vi "Begin.vi"(8 "error in":errorcluster) -> (0 "error out":errorcluster)   [LabVIEW 2019]
doc: "Called before other user functions, this VI is expected to open initial I/O refnums, load in file data, and do all program initialization. Notice that the <B>error out</B> terminal is simply used for data flow. Wiring it to other structures or subVIs ensures that this VI runs first."
uses:
  <vilib>/Rock Robotics/SystemInterfaces/i2clib/i2c_bus.ctl
  <vilib>/Rock Robotics/WPI/DriverStation/WPI_DriverStationRobotMode2.ctl
  <vilib>/Rock Robotics/WPI/Joystick/WPI_JoystickDeviceEnum.ctl
  <vilib>/Rock Robotics/WPI/SafetyOutput/WPI_SafetyOutputConfigMenu.ctl
  <vilib>/Rock Robotics/WPI/ThirdParty/Phoenix-LabVIEW/Motor Controller/Controls/CTRE_Phoenix_MotorControl_ControlMode.ctl
  <vilib>/Rock Robotics/WPI/ThirdParty/Phoenix-LabVIEW/Motor Controller/Controls/CTRE_Phoenix_MotorControl_FeedbackDevice.ctl
  <vilib>/Rock Robotics/WPI/Solenoid/WPI_SolenoidChannel.ctl
  <vilib>/Rock Robotics/WPI/ThirdParty/Phoenix-LabVIEW/Motor Controller/Controls/CTRE_Phoenix_MotorControl_NeutralMode.ctl
  <vilib>/Rock Robotics/WPI/ThirdParty/REV Robotics/SPARK MAX/Typedef/Spark MAX Motor Type.ctl
  <vilib>/Rock Robotics/WPI/ThirdParty/Phoenix-LabVIEW/Motor Controller/Controls/CTRE_Phoenix_MotorControl_FeedbackDevice_TalonFX.ctl
  <vilib>/Rock Robotics/WPI/ThirdParty/Phoenix-LabVIEW/Motor Controller/Controls/CTRE_Phoenix_MotorControl_VelocityMeasurementPeriod.ctl
  <vilib>/Rock Robotics/SystemInterfaces/DIO/FPGA_DIOChannel.ctl
  <vilib>/Rock Robotics/WPI/ThirdParty/REV Robotics/SPARK MAX/Typedef/Spark MAX Control Type.ctl
  Robot Global Data.vi
  <vilib>/Rock Robotics/Network Tables/NT Write String Array.vi
  <vilib>/Rock Robotics/WPI/Solenoid/WPI_SolenoidOpenDouble.vi
  <vilib>/Rock Robotics/WPI/RobotDrive/WPI_RobotDriveOpen4MotorWithExistingMotors.vi
panel:
  in  "Blue Calibration":cluster{"R":dbl, "G":dbl, "B":dbl}={"R"=0.143, "G"=0.427, "B"=0.429}
  in  "Green Calibration":cluster{"R":dbl, "G":dbl, "B":dbl}={"R"=0.197, "G"=0.561, "B"=0.24}
  in  "Red Calibration":cluster{"R":dbl, "G":dbl, "B":dbl}={"R"=0.561, "G"=0.323, "B"=0.114}
  in  "Yellow Calibration":cluster{"R":dbl, "G":dbl, "B":dbl}={"R"=0.361, "G"=0.524, "B"=0.113}
  in  "I2C Bus":T1
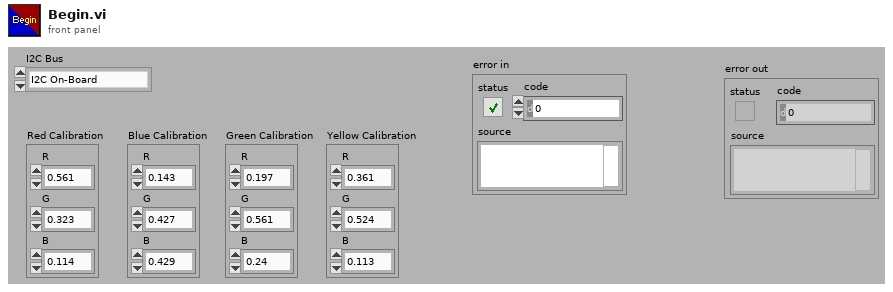
[diagram p1: front panel]
types:
  T1 = typedef "i2c_bus.ctl" = enum16{"I2C On-Board", "I2C MXP", "Invalid"}
  T2 = cluster{"P Gain":dbl, "I Gain":dbl, "D Gain":dbl, "F Gain":dbl, "I Zone":dbl, "Min Output":dbl, "Max Output":dbl}
  T3 = typedef "Spark MAX Motor Type.ctl" = enum16{"Brushed", "Brushless"}
  T4 = typedef "Spark MAX Control Type.ctl" = enum16{"Percent VBus", "Voltage", "Velocity", "Position", "Smart Motion", "Current", "Smart Velocity"}
  T5 = typedef "CTRE_Phoenix_MotorControl_NeutralMode.ctl" = enum8{"EEPROMSetting", "Override to Coast", "Override to Brake"}
  T6 = typedef "WPI_SolenoidChannel.ctl" = enum8{"Solenoid 0", "Solenoid 1", "Solenoid 2", "Solenoid 3", "Solenoid 4", "Solenoid 5", "Solenoid 6", "Solenoid 7", "Invalid"}
  T7 = typedef "FPGA_DIOChannel.ctl" = enum8{"DIO 0", "DIO 1", "DIO 2", "DIO 3", "DIO 4", "DIO 5", "DIO 6", "DIO 7", "DIO 8", "DIO 9", "DIO MXP 0", "DIO MXP 1", "DIO MXP 2", "DIO MXP 3", "DIO MXP 4", "DIO MXP 5", "DIO MXP 6", "DIO MXP 7", "DIO MXP 8", "DIO MXP 9", "DIO MXP 10", "DIO MXP 11", "DIO MXP 12", "DIO MXP 13", "DIO MXP 14", "DIO MXP 15", "SPI Port CS1", "SPI Port CS2", "SPI Port CS3", "SPI Port MISO", "SPI Port MOSI", "Invalid"}
  T8 = typedef "CTRE_Phoenix_MotorControl_VelocityMeasurementPeriod.ctl" = u16
  T9 = typedef "CTRE_Phoenix_MotorControl_FeedbackDevice_TalonFX.ctl" = i8
  T10 = typedef "CTRE_Phoenix_MotorControl_ControlMode.ctl" = u16
  T11 = typedef "CTRE_Phoenix_MotorControl_FeedbackDevice.ctl" = i8
  T12 = typedef "WPI_SafetyOutputConfigMenu.ctl" = enum16{"Enable", "Disable"}
  T13 = typedef "WPI_JoystickDeviceEnum.ctl" = enum16{"USB 0", "USB 1", "USB 2", "USB 3", "USB 4", "USB 5"}
  T14 = typedef "WPI_DriverStationRobotMode2.ctl" = enum16{"Autonomous Disabled", "Autonomous Enabled", "Teleop Disabled", "Teleop Enabled", "Disconnected", "Finish", "Test Disabled", "Test Enabled", "Emergency Stopped"}
  T15 = typedef "Color Sensor V3 DevRef.ctl" = cluster{"I2CDevRef":T16}
  T16 = typedef "WPI_I2CDevRef.ctl" = cluster{"DevStatus":errorcluster, "Device Address":u8, "Handle":i32, "I2C Bus":T1}
  T17 = typedef "WPI_JoystickDevRef.ctl" = cluster{"Device":T13}
  T18 = typedef "WPI_DigitalInputDevRef.ctl" = cluster{"DevStatus":errorcluster, "DIO Channel":T7}
  T19 = typedef "WPI_MotorControlDeviceRef.ctl" = cluster{"DeviceStatus":errorcluster, "Type":T20, "PWM":cluster{"PWM Channel":T21, "DeadBand":T22}, "CAN":cluster{"Device Number":u8, "SetOutput VI Ref":variant, "GetOutput VI Ref":variant, "Enable VI Ref":variant, "Disable VI Ref":variant, "Data":variant}, "Invert":bool, "DIO PWM":cluster{"PWM \"Enable\" Channel":T21, "DIOChannel":T7, "PWM Rate":dbl}}
  T20 = typedef "WPI_MotorControlType.ctl" = enum16{"PWM", "CAN", "DIO PWM"}
  T21 = typedef "FPGA_DIOPWMChannel.ctl" = enum8{"PWM 0", "PWM 1", "PWM 2", "PWM 3", "PWM 4", "PWM 5", "PWM 6", "PWM 7", "PWM 8", "PWM 9", "PWM MXP 0", "PWM MXP 1", "PWM MXP 2", "PWM MXP 3", "PWM MXP 4", "PWM MXP 5", "PWM MXP 6", "PWM MXP 7", "PWM MXP 8", "PWM MXP 9", "Invalid"}
  T22 = typedef "WPI_PWMDeadband.ctl" = cluster{"Name":string, "maxPositivePwm":i32, "minPositivePwm":i32, "centerPwm":i32, "maxNegativePwm":i32, "minNegativePwm":i32, "angularRange":u16}
  T23 = typedef "WPI_SolenoidDevRef.ctl" = cluster{"DevStatus":errorcluster, "Pneumatics Control Module":u8, "Forward Solenoid Channel":T6, "Reverse Solenoid Channel":T6}
  T24 = typedef "WPI_RobotDriveDevRef.ctl" = cluster{"DevStatus":errorcluster, "Motors[]":T19[], "Square Inputs":bool, "Max Output":dbl}
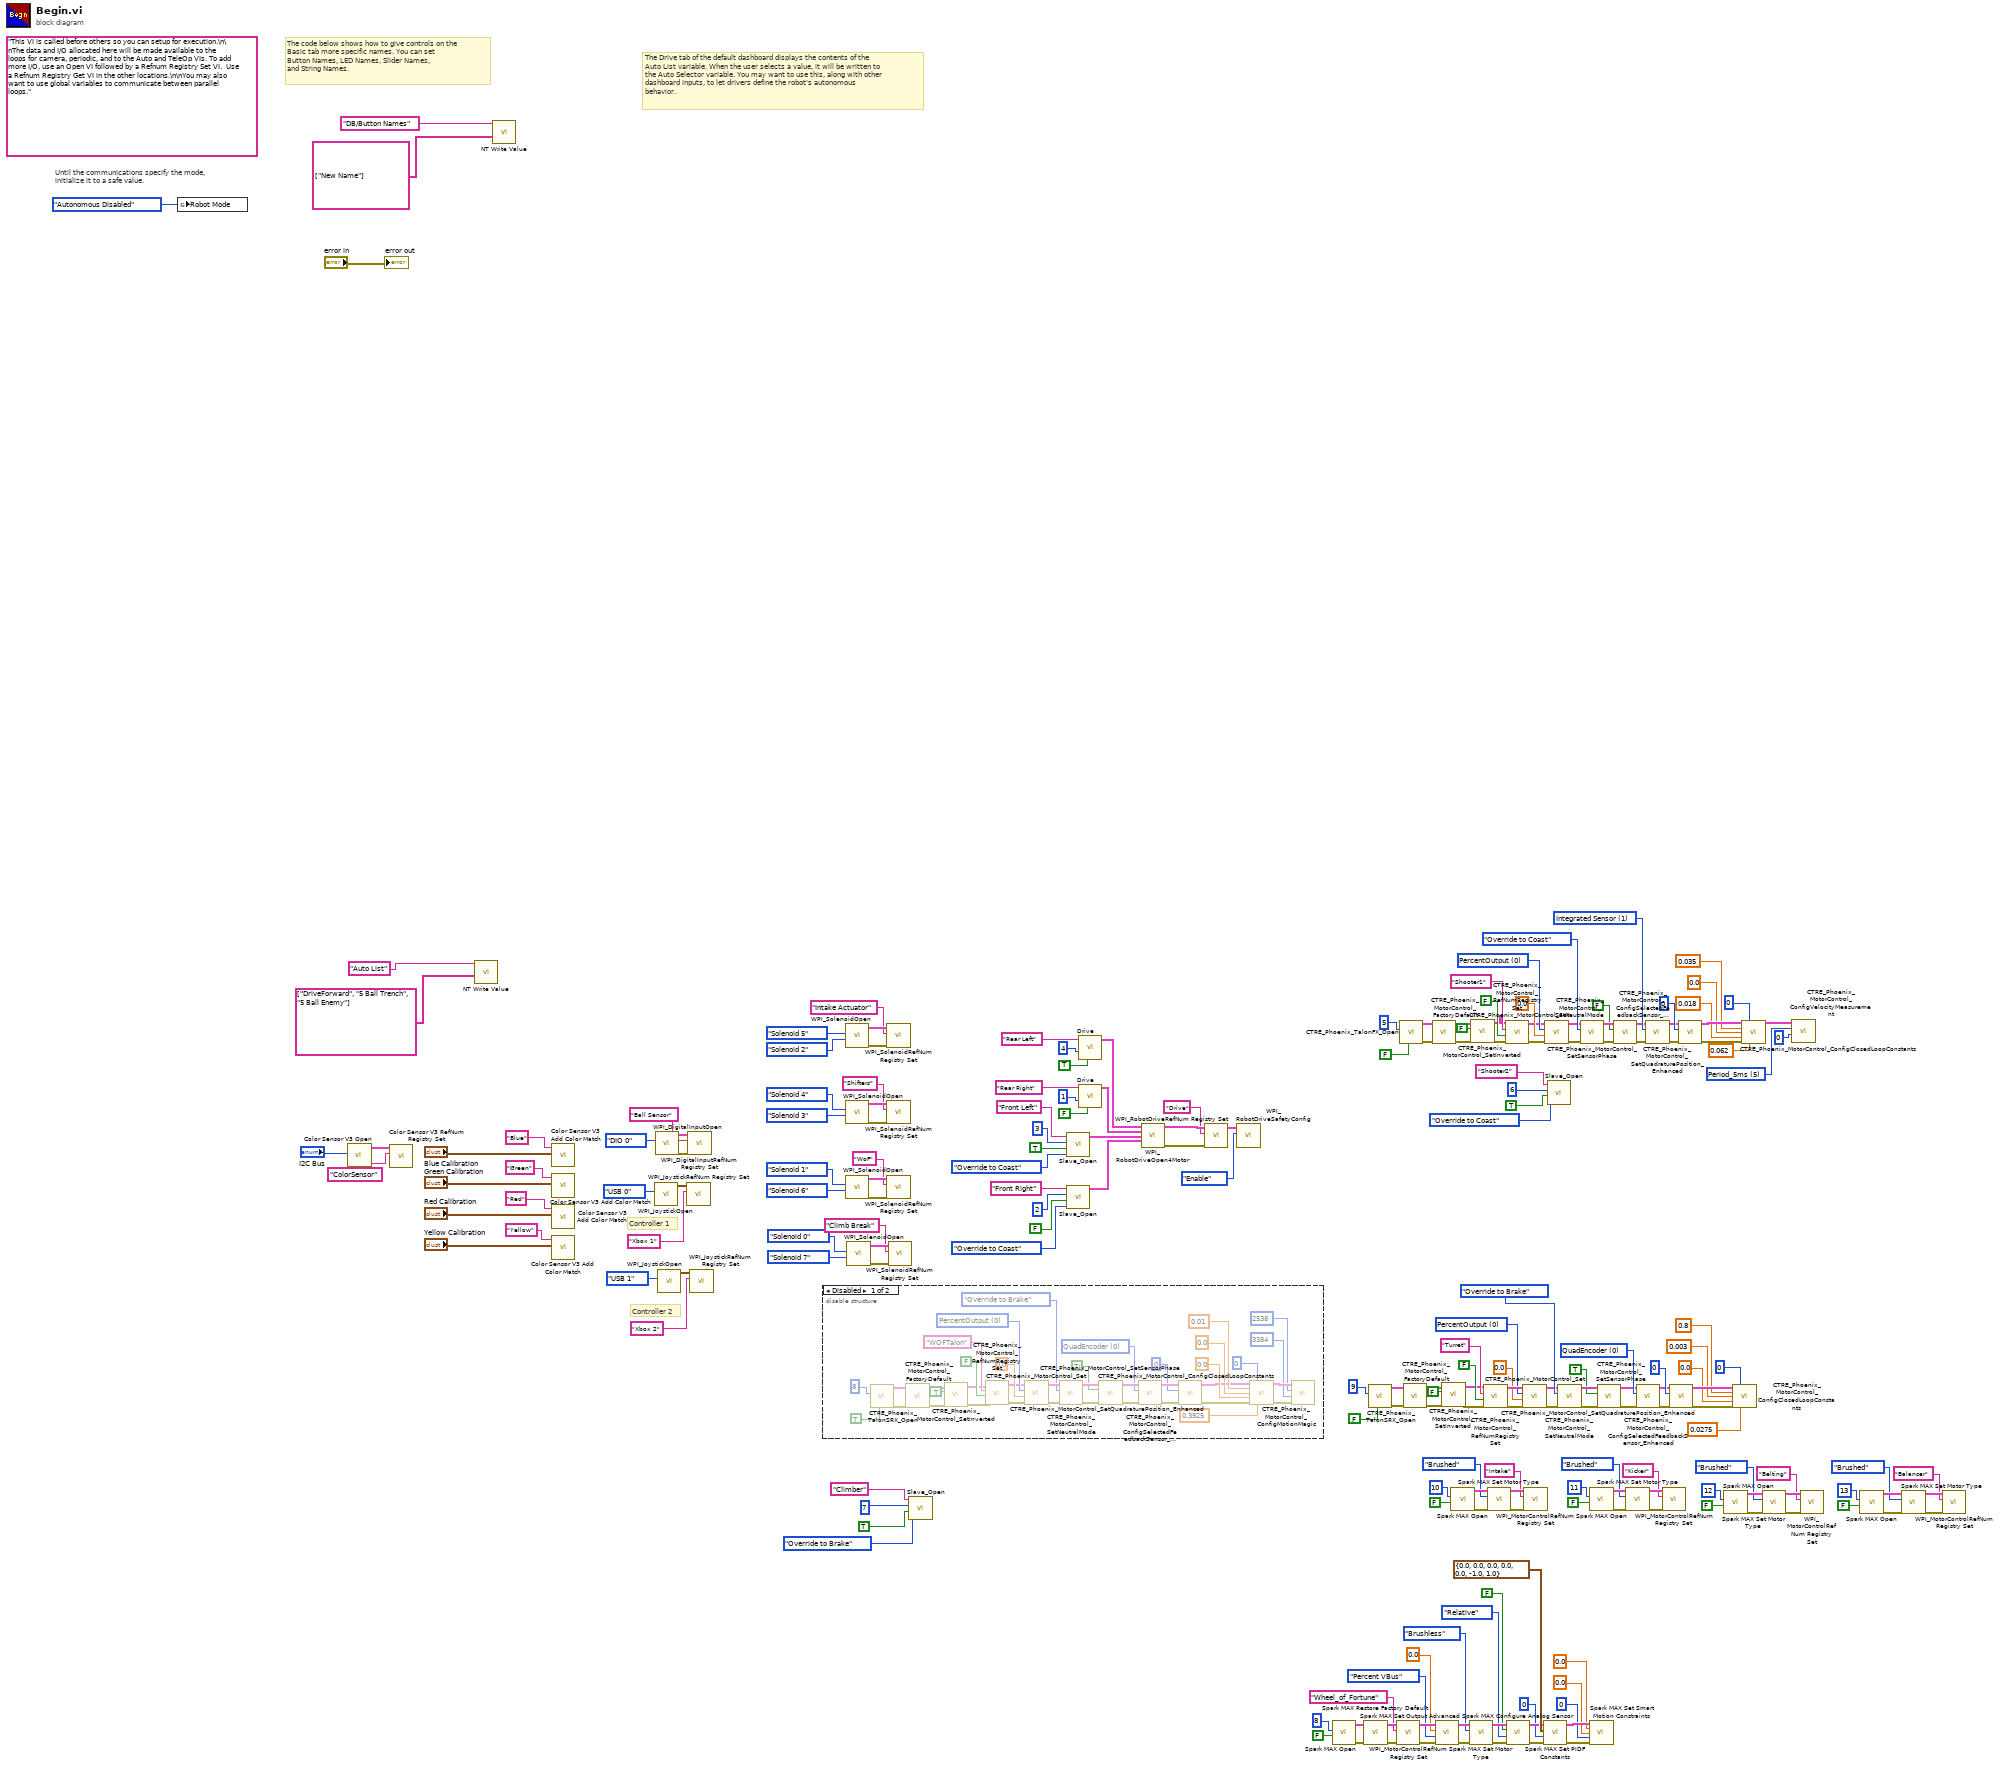
[diagram p0: block diagram]
diagram:
  w123 = T8 5 items=["Period_1ms"=1, "Period_2ms"=2, "Period_5ms"=5, "Period_10ms"=10, "Period_20ms"=20, "Period_25ms"=25, "Period_50ms"=50, "Period_100ms"=100] ("Velocity Measurement Period")
  w113 = T9 1 items=["Integrated Sensor"=1, "Sensor Sum (S0 + S1)"=9, "Sensor Difference (D0 - D1)"=10, "Remote Source 0"=11, "Remote Source 1"=12, "None"=14, "Software Emulated"=15] ("Talon FX Feedback Device")
  w111 = T10 0 items=["PercentOutput"=0, "Position"=1, "Velocity"=2, "Current"=3, "Follower"=5, "MotionProfile"=6, "MotionMagic"=7, "MotionProfileArc"=10, "Disabled"=15] ("Control Mode")
  w166 = T11 0 items=["None"=-1, "QuadEncoder"=0, "Analog"=2, "Tachometer"=4, "Pulse Width Encoded Position"=8, "Sensor Sum (S0 + S1)"=9, "Sensor Difference (D0 - D1)"=10, "Remote Source 0"=11, "Remote Source 1"=12, "Software Emulated"=15] ("Feedback Device")
  w171 = T10 0 items=["PercentOutput"=0, "Position"=1, "Velocity"=2, "Current"=3, "Follower"=5, "MotionProfile"=6, "MotionMagic"=7, "MotionMagicArc"=8, "MotionProfileArc"=10, "Disabled"=15] ("Control Mode")
  (unwired) "This VI is called before others so you can setup for execution.\n\nThe data and I/O allocated here will be made available to the loops for camera, periodic, and to the Auto and TeleOp VIs. To add more I/O, use an Open VI followed by a Refnum Registry Set VI.  Use a Refnum Registry Get VI in the other locations.\n\nYou may also want to use global variables to communicate between parallel loops."
  # "Controller 2"
  # "Controller 1"
  # "The Drive tab of the default dashboard displays the contents of the\nAuto List variable. When the user selects a value, it will be written to\nthe Auto Selector variable. You may want to use this, along with other\ndashboard inputs, to let drivers define the robot's autonomous\nbehavior."
  # "The code below shows how to give controls on the\nBasic tab more specific names. You can set\nButton Names, LED Names, Slider Names,\nand String Names."
  # "Until the communications specify the mode,\ninitialize it to a safe value."
  n1 = global write "Robot Global Data.vi" "Robot Mode"(WPI_DriverStationRobotMode2."Autonomous Disabled" ("Robot Mode")) -> ()
  n2 = call <vilib>:"Color Sensor V3 Open.vi"("I2C Bus"="I2C Bus") -> ("ColorSensorDevRef"=w190:T15)  [unwired: 9 in, 1 out]
  n3 = call <vilib>:"Color Sensor V3 RefNum Registry Set.vi"("refnum name"="ColorSensor", "ColorSensorDevRef"=w190) -> ()  [unwired: 8 in, 2 out]
  n4 = call-poly <vilib>:"NT Write Value.vi"("String Array"=string[] ["DriveForward", "5 Ball Trench", "5 Ball Enemy"], "Name"="Auto List") -> ()  [unwired: 9 in, 1 out]
  n5 = call-poly <vilib>:"NT Write Value.vi"("String Array"=string[] ["New Name"], "Name"="DB/Button Names") -> ()  [unwired: 9 in, 1 out]
  n6 = call <vilib>:"Color Sensor V3 Add Color Match.vi"("Color"="Blue Calibration", "Name"="Blue") -> ()  [unwired: 10 in]
  n7 = call <vilib>:"Color Sensor V3 Add Color Match.vi"("Color"="Green Calibration", "Name"="Green") -> ()  [unwired: 10 in]
  n8 = call <vilib>:"Color Sensor V3 Add Color Match.vi"("Color"="Red Calibration", "Name"="Red") -> ()  [unwired: 10 in]
  n9 = call <vilib>:"Color Sensor V3 Add Color Match.vi"("Color"="Yellow Calibration", "Name"="Yellow") -> ()  [unwired: 10 in]
  n10 = call <vilib>:"WPI_JoystickOpen.vi"("JoystickDevice"=WPI_JoystickDeviceEnum."USB 0") -> ("JoystickDevRef"=w206:T17)  [unwired: 10 in]
  n11 = call <vilib>:"WPI_DigitalInputOpen.vi"("DIO Channel"=FPGA_DIOChannel."DIO 0") -> ("error out"=w94:errorcluster, "DigitalInputDevRef"=w93:T18)  [unwired: 9 in]
  n12 = call <vilib>:"WPI_JoystickOpen.vi"("JoystickDevice"=WPI_JoystickDeviceEnum."USB 1") -> ("JoystickDevRef"=w187:T17)  [unwired: 10 in]
  n13 = call <vilib>:"WPI_JoystickRefNum Registry Set.vi"("refnum name"="Xbox 1", "JoystickDevRef"=w206) -> ()  [unwired: 8 in, 2 out]
  n14 = call <vilib>:"WPI_DigitalInputRefNum Registry Set.vi"("error in (no error)"=w94, "refnum name"="Ball Sensor", "DigitalInputDevRef"=w93) -> ()  [unwired: 7 in, 2 out]
  n15 = call <vilib>:"WPI_JoystickRefNum Registry Set.vi"("refnum name"="Xbox 2", "JoystickDevRef"=w187) -> ()  [unwired: 8 in, 2 out]
  n16 = disable-structure shown="Disabled" {
    frame Disabled {
      w235 = T11 0 items=["None"=-1, "QuadEncoder"=0, "Analog"=2, "Tachometer"=4, "Pulse Width Encoded Position"=8, "Sensor Sum (S0 + S1)"=9, "Sensor Difference (D0 - D1)"=10, "Remote Source 0"=11, "Remote Source 1"=12, "Software Emulated"=15] ("Feedback Device")
      w230 = T10 0 items=["PercentOutput"=0, "Position"=1, "Velocity"=2, "Current"=3, "Follower"=5, "MotionProfile"=6, "MotionMagic"=7, "MotionMagicArc"=8, "MotionProfileArc"=10, "Disabled"=15] ("Control Mode")
      n17 = call <vilib>:"CTRE_Phoenix_TalonSRX_Open.vi"("Invert"=TRUE, "Device Number"=u8 8) -> ("error out"=w214:errorcluster, "CAN Talon SRX Ref"=w215:T19)  [unwired: 8 in]
      n18 = call <vilib>:"CTRE_Phoenix_MotorControl_FactoryDefault.vi"("error in"=w214, "PhoenixMotorControlDevRef"=w215) -> ("error out"=w213:errorcluster, "PhoenixMotorControlDevRef"=w212:T19)  [unwired: 8 in]
      n19 = call <vilib>:"CTRE_Phoenix_MotorControl_SetInverted.vi"("error in (no error)"=w213, "Invert?"=TRUE, "PhoenixMotorControlDevRef"=w212) -> ("error out"=w209:errorcluster, "PhoenixMotorControlDevRef"=w210:T19)  [unwired: 7 in]
      n20 = call <vilib>:"CTRE_Phoenix_MotorControl_RefNumRegistrySet.vi"("error in (no error)"=w209, "Test Mode Only"=FALSE, "refnum name"="WOFTalon", "PhoenixMotorControlDevRef"=w210) -> ("error out"=w228:errorcluster, "PhoenixMotorControlDevRef"=w229:T19)  [unwired: 6 in]
      n21 = call <vilib>:"CTRE_Phoenix_MotorControl_Set.vi"("error in (no error)"=w228, "Output"=0.0, "Control Mode"=w230, "PhoenixMotorControlDevRef"=w229) -> ("error out"=w239:errorcluster, "PhoenixMotorControlDevRef"=w243:T19)  [unwired: 6 in]
      n22 = call <vilib>:"CTRE_Phoenix_MotorControl_SetNeutralMode.vi"("error in (no error)"=w239, "Motor Control Neutral Mode"=CTRE_Phoenix_MotorControl_NeutralMode."Override to Brake", "PhoenixMotorControlDevRef"=w243) -> ("error out"=w241:errorcluster, "PhoenixMotorControlDevRef"=w240:T19)  [unwired: 7 in]
      n23 = call <vilib>:"CTRE_Phoenix_MotorControl_SetSensorPhase.vi"("error in (no error)"=w241, "PhaseSensor"=TRUE, "PhoenixMotorControlDevRef"=w240) -> ("error out"=w237:errorcluster, "PhoenixMotorControlDevRef"=w236:T19)  [unwired: 7 in]
      n24 = call <vilib>:"CTRE_Phoenix_MotorControl_ConfigSelectedFeedbackSensor_Enhanced.vi"("error in (no error)"=w237, "Feedback Device"=w235, "PhoenixMotorControlDevRef"=w236) -> ("error out"=w233:errorcluster, "PhoenixMotorControlDevRef"=w234:T19)  [unwired: 7 in]
      n25 = call <vilib>:"CTRE_Phoenix_MotorControl_SetQuadraturePosition_Enhanced.vi"("error in (no error)"=w233, "New Position"=0, "PhoenixMotorControlDevRef"=w234) -> ("error out"=w216:errorcluster, "PhoenixMotorControlDevRef"=w217:T19)  [unwired: 7 in]
      n26 = call <vilib>:"CTRE_Phoenix_MotorControl_ConfigClosedLoopConstants.vi"("PhoenixMotorControlDevRef"=w217, "slotIdx"=0, "P"=0.01, "I"=0.0, "D"=0.0, "error in (no error)"=w216, "F"=0.3925) -> ("PhoenixMotorControlDevRef"=w225:T19, "error out"=w226:errorcluster)  [unwired: 7 in]
      n27 = call <vilib>:"CTRE_Phoenix_MotorControl_ConfigMotionMagic.vi"("error in (no error)"=w226, "Acceleration"=3384, "Cruise Velocity"=2538, "PhoenixMotorControlDevRef"=w225) -> ()  [unwired: 6 in, 2 out]
    }
    frame Enabled {
    }
  }
  n28 = call-poly <vilib>:"WPI_SolenoidOpen.vi"("Reverse Solenoid Channel"=WPI_SolenoidChannel."Solenoid 2", "Forward Solenoid Channel"=WPI_SolenoidChannel."Solenoid 5") -> ("error out"=w81:errorcluster, "SolenoidDevRef"=w80:T23)  [unwired: 8 in]
  n29 = call-poly <vilib>:"WPI_SolenoidOpen.vi"("Reverse Solenoid Channel"=WPI_SolenoidChannel."Solenoid 3", "Forward Solenoid Channel"=WPI_SolenoidChannel."Solenoid 4") -> ("error out"=w152:errorcluster, "SolenoidDevRef"=w151:T23)  [unwired: 8 in]
  n30 = call-poly <vilib>:"WPI_SolenoidOpen.vi"("Reverse Solenoid Channel"=WPI_SolenoidChannel."Solenoid 6", "Forward Solenoid Channel"=WPI_SolenoidChannel."Solenoid 1") -> ("error out"=w90:errorcluster, "SolenoidDevRef"=w89:T23)  [unwired: 8 in]
  n31 = call-poly <vilib>:"WPI_SolenoidOpen.vi"("Reverse Solenoid Channel"=WPI_SolenoidChannel."Solenoid 7", "Forward Solenoid Channel"=WPI_SolenoidChannel."Solenoid 0") -> ("error out"=w86:errorcluster, "SolenoidDevRef"=w85:T23)  [unwired: 8 in]
  n32 = call <vilib>:"WPI_SolenoidRefNum Registry Set.vi"("error in (no error)"=w81, "refnum name"="Intake Actuator", "SolenoidDevRef"=w80) -> ()  [unwired: 7 in, 2 out]
  n33 = call <vilib>:"WPI_SolenoidRefNum Registry Set.vi"("error in (no error)"=w152, "refnum name"="Shifters", "SolenoidDevRef"=w151) -> ()  [unwired: 7 in, 2 out]
  n34 = call <vilib>:"WPI_SolenoidRefNum Registry Set.vi"("error in (no error)"=w90, "refnum name"="WoF", "SolenoidDevRef"=w89) -> ()  [unwired: 7 in, 2 out]
  n35 = call <vilib>:"WPI_SolenoidRefNum Registry Set.vi"("error in (no error)"=w86, "refnum name"="Climb Break", "SolenoidDevRef"=w85) -> ()  [unwired: 7 in, 2 out]
  n36 = call "Slave_Open.vi"("Motor Control Neutral Mode"=CTRE_Phoenix_MotorControl_NeutralMode."Override to Brake", "Invert"=TRUE, "Device Number"=u8 7, "Motor Name"="Climber" ("refnum name")) -> ()  [unwired: 7 in, 1 out]
  n37 = call "Slave_Open.vi"("Motor Control Neutral Mode"=CTRE_Phoenix_MotorControl_NeutralMode."Override to Coast", "Invert"=TRUE, "Device Number"=u8 3, "Motor Name"="Front Left" ("refnum name")) -> ("PhoenixMotorControlDevRef"=w47:T19)  [unwired: 7 in]
  n38 = call "Slave_Open.vi"("Motor Control Neutral Mode"=CTRE_Phoenix_MotorControl_NeutralMode."Override to Coast", "Invert"=FALSE, "Device Number"=u8 2, "Motor Name"="Front Right" ("refnum name")) -> ("PhoenixMotorControlDevRef"=w46:T19)  [unwired: 7 in]
  n39 = call "Drive.vi"("Invert"=TRUE, "Device Number"=u8 4, "Motor Name"="Rear Left" ("refnum name")) -> ("Motor Out"=w153:T19)  [unwired: 8 in]
  n40 = call "Drive.vi"("Invert"=FALSE, "Device Number"=u8 1, "Motor Name"="Rear Right" ("refnum name")) -> ("Motor Out"=w68:T19)  [unwired: 8 in]
  n41 = call-poly <vilib>:"WPI_RobotDriveOpen4Motor.vi"("Rear Left Motor Dev Ref"=w153, "Rear Right Motor Dev Ref"=w68, "Front Left Motor Dev Ref"=w47, "Front Right Motor Dev Ref"=w46) -> ("RobotDriveDevRef"=w185:T24, "error out"=w183:errorcluster)  [unwired: 10 in]
  n42 = call <vilib>:"WPI_RobotDriveRefNum Registry Set.vi"("error in (no error)"=w183, "refnum name"="Drive", "RobotDriveDevRef"=w185) -> ("RobotDriveDevRef"=w182:T24)  [unwired: 1 in, 7 out]
  n43 = call <vilib>:"WPI_RobotDriveSafetyConfig.vi"("mode"=WPI_SafetyOutputConfigMenu."Enable", "RobotDriveDevRef"=w182) -> ()  [unwired: 8 in, 2 out]
  n44 = call <vilib>:"Spark MAX Open.vi"("Invert"=FALSE, "Device Number"=u8 8) -> ("error out"=w33:errorcluster, "MotorControlDeviceRef"=w32:T19)  [unwired: 8 in]
  n45 = call <vilib>:"Spark MAX Restore Factory Default.vi"("error in"=w33, "MotorControlDeviceRef"=w32) -> ("error out"=w23:errorcluster, "MotorControlDeviceRef"=w22:T19)  [unwired: 8 in]
  n46 = call <vilib>:"CTRE_Phoenix_TalonSRX_Open.vi"("Invert"=FALSE, "Device Number"=u8 9) -> ("error out"=w55:errorcluster, "CAN Talon SRX Ref"=w54:T19)  [unwired: 8 in]
  n47 = call <vilib>:"WPI_MotorControlRefNum Registry Set.vi"("error in (no error)"=w23, "refnum name"="Wheel_of_Fortune", "MotorControlDevRef"=w22) -> ("error out"=w21:errorcluster, "MotorControlDevRef"=w20:T19)  [unwired: 7 in]
  n48 = call <vilib>:"CTRE_Phoenix_TalonFX_Open.vi"("Invert"=FALSE, "Device Number"=u8 5) -> ("error out"=w62:errorcluster, "CAN Talon SRX Ref"=w61:T19)  [unwired: 8 in]
  n49 = call <vilib>:"CTRE_Phoenix_MotorControl_FactoryDefault.vi"("error in"=w55, "PhoenixMotorControlDevRef"=w54) -> ("error out"=w60:errorcluster, "PhoenixMotorControlDevRef"=w59:T19)  [unwired: 8 in]
  n50 = call <vilib>:"CTRE_Phoenix_MotorControl_FactoryDefault.vi"("error in"=w62, "PhoenixMotorControlDevRef"=w61) -> ("error out"=w67:errorcluster, "PhoenixMotorControlDevRef"=w66:T19)  [unwired: 8 in]
  n51 = call <vilib>:"Spark MAX Set Output Advanced.vi"("error in (no error)"=w21, "Control Mode"=Spark_MAX_Control_Type."Percent VBus", "Setpoint"=0.0, "MotorControlDevRef"=w20) -> ("error out"=w17:errorcluster, "MotorControlDevRef"=w16:T19)  [unwired: 6 in]
  n52 = call <vilib>:"CTRE_Phoenix_MotorControl_SetInverted.vi"("error in (no error)"=w60, "Invert?"=FALSE, "PhoenixMotorControlDevRef"=w59) -> ("error out"=w56:errorcluster, "PhoenixMotorControlDevRef"=w57:T19)  [unwired: 7 in]
  n53 = call <vilib>:"Spark MAX Open.vi"("Invert"=FALSE, "Device Number"=u8 10) -> ("error out"=w147:errorcluster, "MotorControlDeviceRef"=w148:T19)  [unwired: 8 in]
  n54 = call <vilib>:"Spark MAX Set Motor Type.vi"("error in (no error)"=w17, "Motor Type"=Spark_MAX_Motor_Type."Brushless", "MotorControlDevRef"=w16) -> ("error out"=w13:errorcluster, "MotorControlDeviceRef"=w14:T19)  [unwired: 7 in]
  n55 = call <vilib>:"CTRE_Phoenix_MotorControl_SetInverted.vi"("error in (no error)"=w67, "Invert?"=FALSE, "PhoenixMotorControlDevRef"=w66) -> ("error out"=w63:errorcluster, "PhoenixMotorControlDevRef"=w64:T19)  [unwired: 7 in]
  n56 = call <vilib>:"CTRE_Phoenix_MotorControl_RefNumRegistrySet.vi"("error in (no error)"=w56, "Test Mode Only"=FALSE, "refnum name"="Turret", "PhoenixMotorControlDevRef"=w57) -> ("error out"=w173:errorcluster, "PhoenixMotorControlDevRef"=w172:T19)  [unwired: 6 in]
  n57 = call <vilib>:"Spark MAX Set Motor Type.vi"("error in (no error)"=w147, "Motor Type"=Spark_MAX_Motor_Type."Brushed", "MotorControlDevRef"=w148) -> ("error out"=w145:errorcluster, "MotorControlDeviceRef"=w144:T19)  [unwired: 7 in]
  n58 = call <vilib>:"CTRE_Phoenix_MotorControl_RefNumRegistrySet.vi"("error in (no error)"=w63, "Test Mode Only"=FALSE, "refnum name"="Shooter1", "PhoenixMotorControlDevRef"=w64) -> ("error out"=w100:errorcluster, "PhoenixMotorControlDevRef"=w101:T19)  [unwired: 6 in]
  n59 = call <vilib>:"Spark MAX Configure Analog Sensor.vi"("error in (no error)"=w13, "Sensor Mode (Absolute)"=enum16{"Absolute", "Relative"}."Relative", "Inverted (F)"=FALSE, "MotorControlDeviceRef in"=w14) -> ("error out"=w6:errorcluster, "MotorControlDeviceRef"=w7:T19)  [unwired: 6 in]
  n60 = call <vilib>:"CTRE_Phoenix_MotorControl_Set.vi"("error in (no error)"=w173, "Output"=0.0, "Control Mode"=w171, "PhoenixMotorControlDevRef"=w172) -> ("error out"=w163:errorcluster, "PhoenixMotorControlDevRef"=w159:T19)  [unwired: 6 in]
  n61 = call <vilib>:"WPI_MotorControlRefNum Registry Set.vi"("error in (no error)"=w145, "refnum name"="Intake", "MotorControlDevRef"=w144) -> ()  [unwired: 7 in, 2 out]
  n62 = call <vilib>:"Spark MAX Set PIDF Constants.vi"("error in"=w6, "PIDF Slot"=0, "PID Constants"=T2 {"P Gain"=0.0, "I Gain"=0.0, "D Gain"=0.0, "F Gain"=0.0, "I Zone"=0.0, "Min Output"=-1.0, "Max Output"=1.0}, "MotorControlDeviceRef"=w7) -> ("error out"=w5:errorcluster, "MotorControlDeviceRef"=w8:T19)  [unwired: 6 in]
  n63 = call <vilib>:"CTRE_Phoenix_MotorControl_Set.vi"("error in (no error)"=w100, "Output"=0.0, "Control Mode"=w111, "PhoenixMotorControlDevRef"=w101) -> ("error out"=w102:errorcluster, "PhoenixMotorControlDevRef"=w103:T19)  [unwired: 6 in]
  n64 = call "Slave_Open.vi"("Motor Control Neutral Mode"=CTRE_Phoenix_MotorControl_NeutralMode."Override to Coast", "Invert"=TRUE, "Device Number"=u8 6, "Motor Name"="Shooter2" ("refnum name")) -> ()  [unwired: 7 in, 1 out]
  n65 = call <vilib>:"CTRE_Phoenix_MotorControl_SetNeutralMode.vi"("error in (no error)"=w163, "Motor Control Neutral Mode"=CTRE_Phoenix_MotorControl_NeutralMode."Override to Brake", "PhoenixMotorControlDevRef"=w159) -> ("error out"=w161:errorcluster, "PhoenixMotorControlDevRef"=w162:T19)  [unwired: 7 in]
  n66 = call <vilib>:"CTRE_Phoenix_MotorControl_SetNeutralMode.vi"("error in (no error)"=w102, "Motor Control Neutral Mode"=CTRE_Phoenix_MotorControl_NeutralMode."Override to Coast", "PhoenixMotorControlDevRef"=w103) -> ("error out"=w104:errorcluster, "PhoenixMotorControlDevRef"=w105:T19)  [unwired: 7 in]
  n67 = call <vilib>:"Spark MAX Open.vi"("Invert"=FALSE, "Device Number"=u8 11) -> ("error out"=w131:errorcluster, "MotorControlDeviceRef"=w132:T19)  [unwired: 8 in]
  n68 = call <vilib>:"Spark MAX Set Smart Motion Constraints.vi"("MotorControlDeviceRef"=w8, "Max Velocity"=0.0, "Max Acceleration"=0.0, "PIDF Slot (0)"=0, "error in"=w5) -> ()  [unwired: 9 in, 2 out]
  n69 = call <vilib>:"CTRE_Phoenix_MotorControl_SetSensorPhase.vi"("error in (no error)"=w161, "PhaseSensor"=TRUE, "PhoenixMotorControlDevRef"=w162) -> ("error out"=w164:errorcluster, "PhoenixMotorControlDevRef"=w165:T19)  [unwired: 7 in]
  n70 = call <vilib>:"CTRE_Phoenix_MotorControl_SetSensorPhase.vi"("error in (no error)"=w104, "PhaseSensor"=FALSE, "PhoenixMotorControlDevRef"=w105) -> ("error out"=w106:errorcluster, "PhoenixMotorControlDevRef"=w107:T19)  [unwired: 7 in]
  n71 = call <vilib>:"Spark MAX Set Motor Type.vi"("error in (no error)"=w131, "Motor Type"=Spark_MAX_Motor_Type."Brushed", "MotorControlDevRef"=w132) -> ("error out"=w129:errorcluster, "MotorControlDeviceRef"=w128:T19)  [unwired: 7 in]
  n72 = call <vilib>:"CTRE_Phoenix_MotorControl_ConfigSelectedFeedbackSensor_Enhanced.vi"("error in (no error)"=w164, "Feedback Device"=w166, "PhoenixMotorControlDevRef"=w165) -> ("error out"=w168:errorcluster, "PhoenixMotorControlDevRef"=w167:T19)  [unwired: 7 in]
  n73 = call <vilib>:"CTRE_Phoenix_MotorControl_ConfigSelectedFeedbackSensor_TalonFX.vi"("error in (no error)"=w106, "Talon FX Feedback Device"=w113, "PhoenixMotorControlDevRef"=w107) -> ("error out"=w108:errorcluster, "PhoenixMotorControlDevRef"=w109:T19)  [unwired: 7 in]
  n74 = call <vilib>:"WPI_MotorControlRefNum Registry Set.vi"("error in (no error)"=w129, "refnum name"="Kicker", "MotorControlDevRef"=w128) -> ()  [unwired: 7 in, 2 out]
  n75 = call <vilib>:"CTRE_Phoenix_MotorControl_SetQuadraturePosition_Enhanced.vi"("error in (no error)"=w168, "New Position"=0, "PhoenixMotorControlDevRef"=w167) -> ("error out"=w180:errorcluster, "PhoenixMotorControlDevRef"=w179:T19)  [unwired: 7 in]
  n76 = call <vilib>:"CTRE_Phoenix_MotorControl_SetQuadraturePosition_Enhanced.vi"("error in (no error)"=w108, "New Position"=0, "PhoenixMotorControlDevRef"=w109) -> ("error out"=w122:errorcluster, "PhoenixMotorControlDevRef"=w121:T19)  [unwired: 7 in]
  n77 = call <vilib>:"Spark MAX Open.vi"("Invert"=FALSE, "Device Number"=u8 12) -> ("error out"=w139:errorcluster, "MotorControlDeviceRef"=w140:T19)  [unwired: 8 in]
  n78 = call <vilib>:"CTRE_Phoenix_MotorControl_ConfigClosedLoopConstants.vi"("PhoenixMotorControlDevRef"=w179, "slotIdx"=0, "P"=0.8, "I"=0.003, "D"=0.0, "error in (no error)"=w180, "F"=0.0275) -> ()  [unwired: 7 in, 2 out]
  n79 = call <vilib>:"CTRE_Phoenix_MotorControl_ConfigClosedLoopConstants.vi"("PhoenixMotorControlDevRef"=w121, "slotIdx"=0, "P"=0.035, "I"=0.0, "D"=0.018, "error in (no error)"=w122, "F"=0.062) -> ("PhoenixMotorControlDevRef"=w124:T19)  [unwired: 7 in, 1 out]
  n80 = call <vilib>:"Spark MAX Set Motor Type.vi"("error in (no error)"=w139, "Motor Type"=Spark_MAX_Motor_Type."Brushed", "MotorControlDevRef"=w140) -> ("error out"=w137:errorcluster, "MotorControlDeviceRef"=w136:T19)  [unwired: 7 in]
  n81 = call <vilib>:"CTRE_Phoenix_MotorControl_ConfigVelocityMeasurement.vi"("Window Size"=0, "Velocity Measurement Period"=w123, "PhoenixMotorControlDevRef"=w124) -> ()  [unwired: 7 in, 2 out]
  n82 = call <vilib>:"WPI_MotorControlRefNum Registry Set.vi"("error in (no error)"=w137, "refnum name"="Belting", "MotorControlDevRef"=w136) -> ()  [unwired: 7 in, 2 out]
  n83 = call <vilib>:"Spark MAX Open.vi"("Invert"=FALSE, "Device Number"=u8 13) -> ("error out"=w30:errorcluster, "MotorControlDeviceRef"=w31:T19)  [unwired: 8 in]
  n84 = call <vilib>:"Spark MAX Set Motor Type.vi"("error in (no error)"=w30, "Motor Type"=Spark_MAX_Motor_Type."Brushed", "MotorControlDevRef"=w31) -> ("error out"=w28:errorcluster, "MotorControlDeviceRef"=w27:T19)  [unwired: 7 in]
  n85 = call <vilib>:"WPI_MotorControlRefNum Registry Set.vi"("error in (no error)"=w28, "refnum name"="Balancer", "MotorControlDevRef"=w27) -> ()  [unwired: 7 in, 2 out]
  "error out" <- "error in"
